vi "IsProxy.vi"(8 "error in (no error)":errorcluster, 11 "OperationLogger (proxy) in":refnum<class "OperationLogger (proxy).lvclass">) -> (0 "error out":errorcluster, 2 "isProxy?":bool, 3 "OperationLogger (proxy) out":refnum<class "OperationLogger (proxy).lvclass">)   [LabVIEW 2014, in "forcible Proxy.lvlib" / "OperationLogger (proxy).lvclass"]
uses:
  OperationLogger (proxy).lvclass
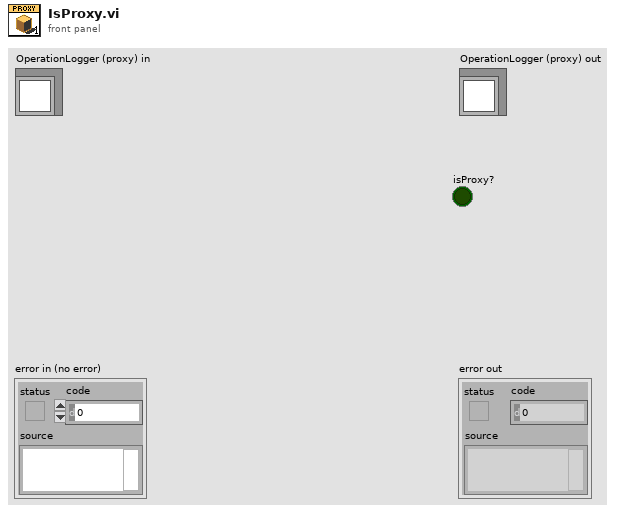
[diagram p1: front panel]
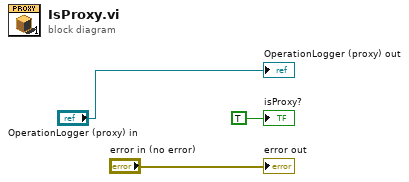
[diagram p0: block diagram]
diagram:
  "error out" <- "error in (no error)"
  "OperationLogger (proxy) out" <- "OperationLogger (proxy) in"
  "isProxy?" <- TRUE ("isProxy?")
